vi "Wait for Registered.vi"(8 "error in (no error)":errorcluster, 9 "ms Timeout (5000)":u32=5000, 11 "User Event Name":string) -> (0 "error out":errorcluster, 1 "ms Elapsed":u32, 3 "User Event":refnum<user-event>)   [LabVIEW 2021, in "UserEvent.lvlib"]
uses:
  UserEvent.lvlib
  <vilib>/Utility/error.llb/Error Cluster From Error Code.vi
  <vilib>/ErrorRing/Error Ring.xnode
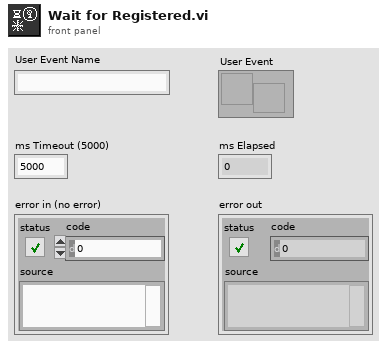
[diagram p1: front panel]
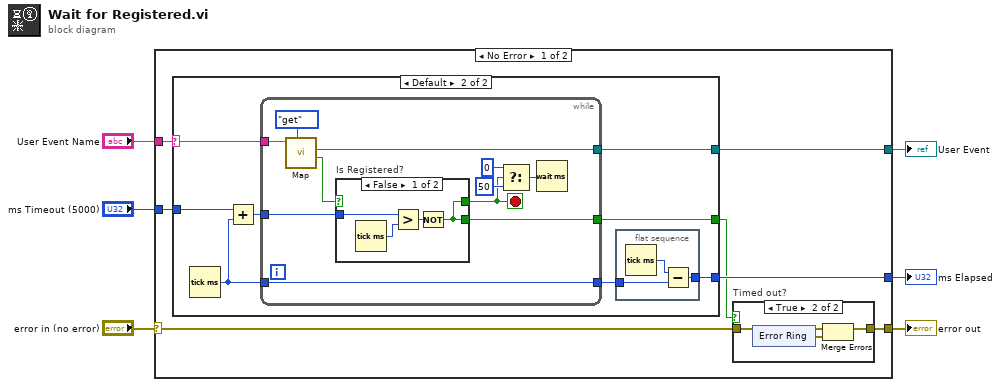
[diagram p0: block diagram]
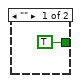
[diagram p2: hidden frame]
diagram:
  n1 = case shown="No Error" "error in (no error)" {
    selector: "error in (no error)" -> [w11 w50]
    tunnel: "User Event Name" -> [w13 _]
    tunnel: [w12 _] -> w5
    tunnel: [w10 w50] -> w3
    tunnel: "ms Timeout (5000)" -> [w9 _]
    tunnel: [w8 _] -> w1
    frame No Error {
      n2 = case shown="Default" w13 {
        selector: w13 -> [_ w22]
        tunnel: [_ w21] -> w12
        tunnel: w9 -> [_ w20]
        tunnel: [_ w19] -> w8
        tunnel: [TRUE w15] -> w7
        frame "" {
        }
        frame Default {
          n3 = Tick Count (ms)() -> (millisecond timer value=w18:u32)
          n4 = Add(x=w20, y=w18) -> (x+y=w16:u32)
          n5 = while {
            tunnel: w22 -> [w35]
            tunnel: [w34] -> w21
            tunnel: [w33] -> w17
            tunnel: w18 -> [w33]
            tunnel: w16 -> [w29]
            tunnel: [w26] -> w15
            stop <- w27 stop-if-true
            n6 = call "Map.vi"("Action"=enum8{"noop", "get", "set", "pop"}."get", "User Event Name"=w35) -> ("Is Registered out"=w28:bool, "User Event out"=w34:refnum<user-event>)  [unwired: 6 in, 2 out]
            n7 = case "Is Registered?" shown="False" w28 {
              selector: w28 -> [_ w41]
              tunnel: w29 -> [w40 _]
              tunnel: [w37 _] -> w26
              tunnel: [w37 w41] -> w27
              frame False {
                n8 = Tick Count (ms)() -> (millisecond timer value=w39:u32)
                n9 = Greater?(x=w40, y=w39) -> (0:w38:bool)
                n10 = Not(x=w38) -> (.not. x?=w37:bool)
              }
              frame True {
              }
            }
            n11 = Select(t=u32 0 ("milliseconds to wait"), s=w27, f=u32 50 ("milliseconds to wait")) -> (s? t:f=w31:u32)
            n12 = Wait (ms)(milliseconds to wait=w31) -> ()  [unwired: 1 out]
          }
          n13 = flat-sequence {
            tunnel: w17 -> [w24]
            tunnel: [w23] -> w19
            frame #0 {
              n14 = Tick Count (ms)() -> (millisecond timer value=w25:u32)
              n15 = Subtract(x=w25, y=w24) -> (x-y=w23:u32)
            }
          }
        }
      }
      n16 = case "Timed out?" shown="True" w7 {
        tunnel: w11 -> [w42 w44]
        tunnel: [w42 w43] -> w10
        frame False {
        }
        frame True {
          n17 = xnode "Error Ring"() -> ("error out"=w45:errorcluster)
          n18 = Merge Errors(w44, w45) -> (w43:errorcluster)
        }
      }
    }
    frame Error {
    }
  }
  "error out" <- w3
  "User Event" <- w5
  "ms Elapsed" <- w1
